vi "subXMLGetSourceItemNames.vi"(11 "Refnum in":refnum<k20>) -> (3 "Names":string[](array[string]))   [LabVIEW 2019, in "SolutionBuilder.lvlib" / "SolutionBuilder.lvclass"]
uses:
  SolutionBuilder.lvclass
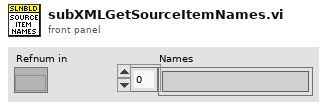
[diagram p1: front panel]
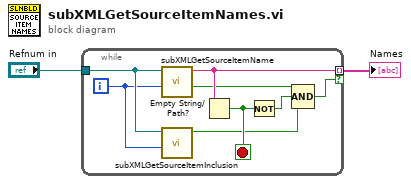
[diagram p0: block diagram]
diagram:
  n1 = while {
    tunnel: [w10] -> w2 mode=indexing if=w5
    tunnel: "Refnum in" -> [w8]
    i -> [w3]
    stop <- w9 stop-if-true
    n2 = call "subXMLGetSourceItemName.vi"("index (1)"=w3, "Refnum in"=w8) -> ("Ref type?"=w4:bool, "source name"=w10:string)  [unwired: 8 in]
    n3 = call "subXMLGetSourceItemInclusion.vi"("index (1)"=w3, "Refnum in"=w8) -> ("Include?"=w6:bool)  [unwired: 9 in]
    n4 = Empty String/Path?(string/path=w10) -> (empty?=w9:bool)
    n5 = Not(x=w9) -> (.not. x?=w7:bool)
    n6 = Compound Arithmetic op=AND(w4, w7, w6) -> (w5:bool)
  }
  "Names" <- w2
